vi "Write Display Settings 2 File.vi"(8 "error in":errorcluster, 11 "State":T6={"ImageSource"=enum."Camera", "IMAQdx Cam"=refnum, "WorkDir"=path "", "Image Name Prefix"="", "ROI"={"Global Rectangle"=[], "Contours"=[]}, "BG Image"=refnum, "Display Image"=refnum, "Display settings"={"Min. Thresh."=0.0, "X"=0.0, "Y"=0.0, "ShowLineout"=FALSE, "ScaleParts"=10, "ShowLegende"=FALSE, "Target Cross"=FALSE, "Centroid Cross"=FALSE, "Target color"=16777226, "Centroid color"=16711680, "calibr. mm/px"=0.0}, "Mask image"=refnum, "ConfigDir"=path "", "Display ref"=refnum, "Saved ROIs"=[], "Selected ROI"="", "Analyze Objects"=[], "Analysis Params"=variant, "Analysis Results"=variant, "Overlays?"=[], "Ref Palette type"=refnum, "Time in Filename?"=TRUE, "Save Report?"=TRUE, "Appl Params"=variant, "Show ZoomBtn?"=TRUE, "Image file"=path ""} {"ROI"."Contours"."Type" items=["No Selection", "Point", "Line", "Rectangle", "Oval", "Polygon", "Freehand Region", "Annulus", "Unused2", "Unused3", "Broken Line", "Freehand Line", "Rotated Rectangle"]}) -> (0 "error out":errorcluster, 3 "file path out":path)   [LabVIEW 2020, in "POLARIS IMAQ Display.xctl"]
doc: "Store some settings of POLARIS IMAQ Display to file. \n[in] State cluster of XControl\nVI maps paramters of interest to dummy controls like ROI, SavedROI, Display settings and calls \n\"save cotrol values.vi\". The dummy contorl must have the same names like dummy controls in Read Display Settings.vi\n\n\nauthor: Alexander Kessler, Helmholtz-Institut-Jena \nmaintainer: Alexander Kessler: alexander.kessler@uni-jena.de\n\n\n\nLicense Agreement for this software:\n\nCopyright (C)\nHelmholtz-Institut-Jena\nFröbelstieg 3\n07743 Jena\nGermany\n\nThis program is free software; you can redistribute it and/or modify it under the terms of the GNU General Public License as published by the Free Software Foundation; either version 2 of the license, or (at your option) any later version.\n\nThis program is distributed in the hope that it will be useful, but WITHOUT ANY WARRANTY; without even the implied warranty of MERCHANTABILITY or FITNESS FOR A PARTICULAR PURPOSE. See the GNU General License for more details (http://www.gnu.org)."
uses:
  POLARIS IMAQ Display.xctl
  State.ctl
  IMAQdx Cam/IMAQdx Cam.lvclass
  Properties/ImageSource.ctl
  <vilib>/vision/Image Controls.llb/IMAQ Image.ctl
  DisplaySettings.ctl
  Named ROI.ctl
  Analyze Classes/Analyze BaseClass/Analyze BaseClass.lvclass
  Palette.ctl
  Utility/POLARIS Vision utility.lvlib
panel:
  in  "Pallete":T1={"Teiler"=1, "Palette Type"=0} {"Teiler" min=1 max=5; "Palette Type" items=["Grayscale", "Binary", "Gradient", "Rainbow", "Temperature", "User Defined"]}
  in  "Zoom":cluster{"X":i32, "Y":i32}
  in  "Image Center":cluster{"X":u32, "Y":u32}
  out "Image":T2(plugin-control)
  in  "Display settings":T3={"Min. Thresh."=0.0, "X"=0.0, "Y"=0.0, "ShowLineout"=FALSE, "ScaleParts"=10, "ShowLegende"=FALSE, "Target Cross"=FALSE, "Centroid Cross"=FALSE, "Target color"=16777226, "Centroid color"=16711680, "calibr. mm/px"=0.0}
  in  "ROI":T4 {"Contours"."Type" items=["No Selection", "Point", "Line", "Rectangle", "Oval", "Polygon", "Freehand Region", "Annulus", "Unused2", "Unused3", "Broken Line", "Freehand Line", "Rotated Rectangle"]}
  in  "Saved ROIs":T5[](array[typedef])
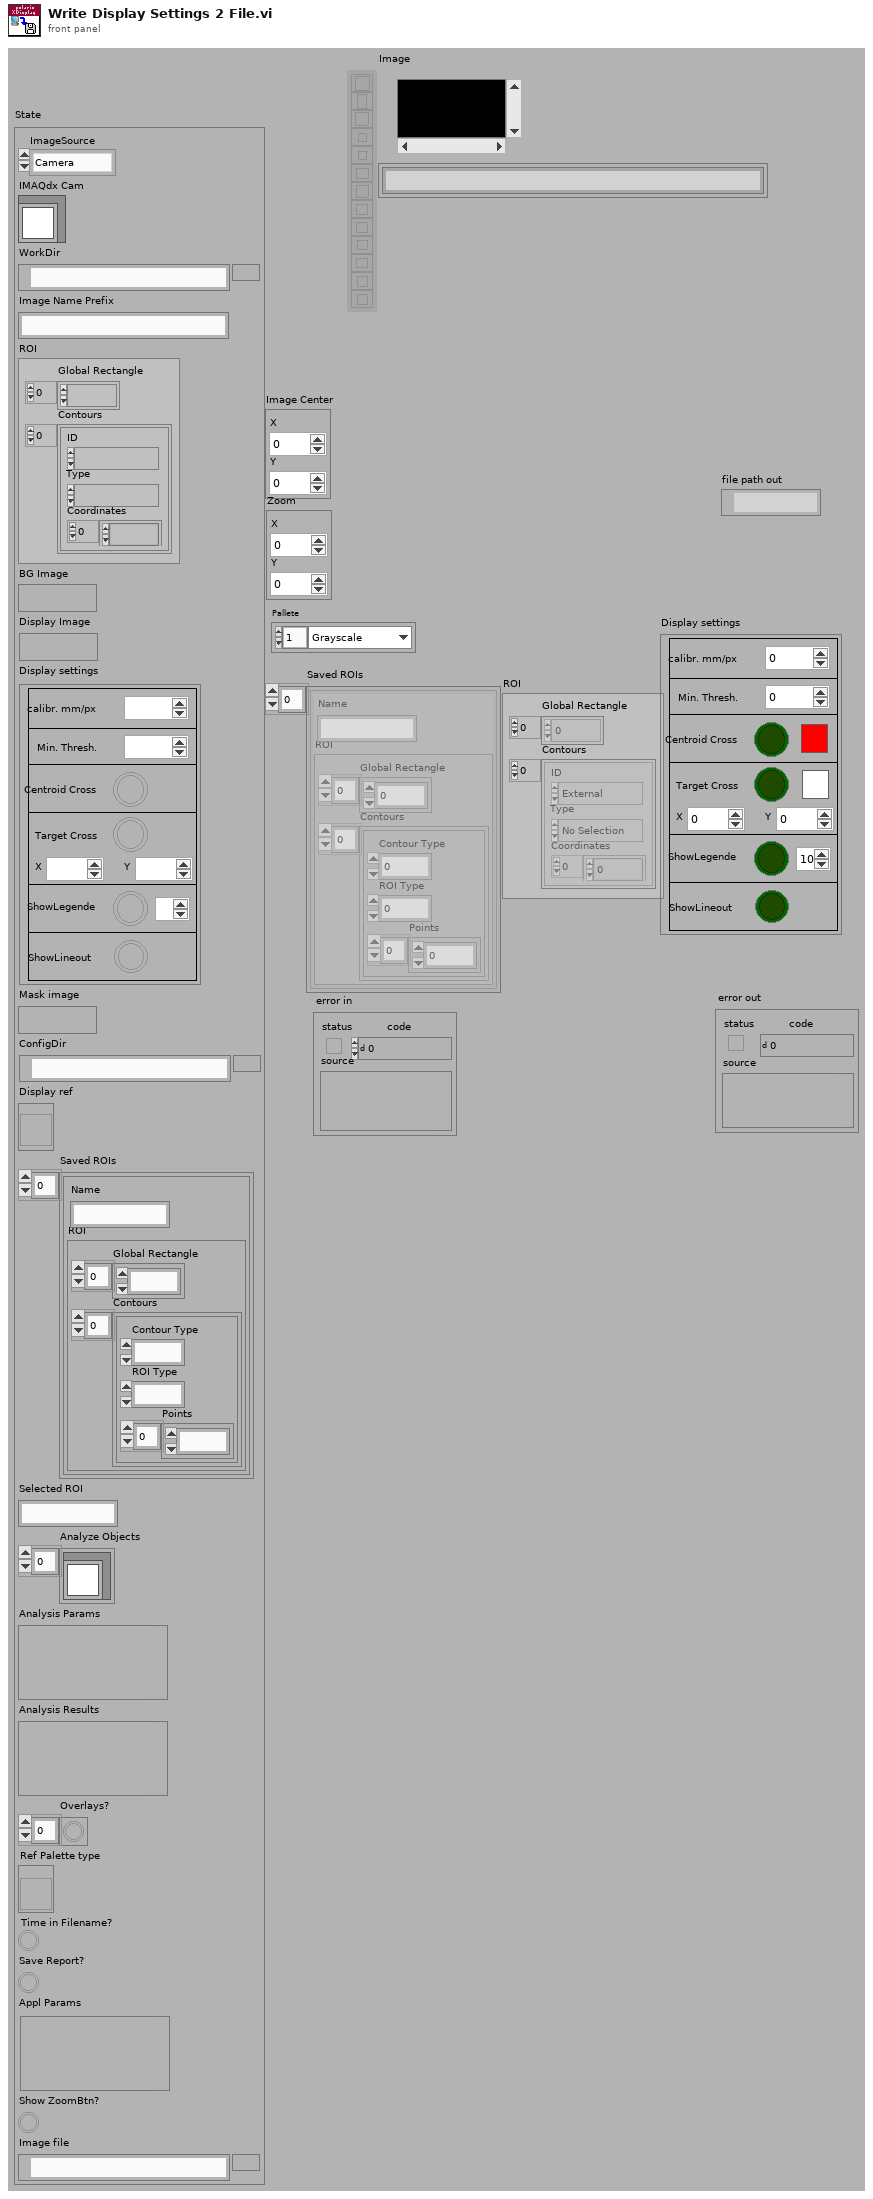
[diagram p1: front panel]
types:
  T1 = typedef "POLARIS IMAQ Display.xctl/Palette.ctl" = cluster{"Teiler":i32, "Palette Type":u32}
  T2 = typedef "IMAQ Image.ctl" = refnum<image>
  T3 = typedef "POLARIS IMAQ Display.xctl/DisplaySettings.ctl" = cluster{"Min. Thresh.":sgl, "X":dbl, "Y":dbl, "ShowLineout":bool, "ScaleParts":i32, "ShowLegende":bool, "Target Cross":bool, "Centroid Cross":bool, "Target color":u32, "Centroid color":u32, "calibr. mm/px":sgl}
  T4 = typedef "ROI Descriptor" = cluster{"Global Rectangle":i32[], "Contours":cluster{"ID":enum32{"External", "Internal"}, "Type":u32, "Coordinates":i32[]}[]}
  T5 = typedef "POLARIS IMAQ Display.xctl/Named ROI.ctl" = cluster{"ROI":cluster{"Global Rectangle":i32[], "Contours":cluster{"Contour Type":u32, "ROI Type":u32, "Points":i32[]}[]}, "Name":string}
  T6 = typedef "POLARIS IMAQ Display.xctl/State.ctl" = cluster{"ImageSource":T7, "IMAQdx Cam":refnum<class "IMAQdx Cam.lvclass">, "WorkDir":path, "Image Name Prefix":string, "ROI":T4, "BG Image":T2, "Display Image":T2, "Display settings":T3, "Mask image":T2, "ConfigDir":path, "Display ref":refnum<vi>, "Saved ROIs":T5[], "Selected ROI":string, "Analyze Objects":refnum<class "Analyze BaseClass.lvclass">[], "Analysis Params":variant, "Analysis Results":variant, "Overlays?":bool[], "Ref Palette type":refnum<vi>, "Time in Filename?":bool, "Save Report?":bool, "Appl Params":variant, "Show ZoomBtn?":bool, "Image file":path}
  T7 = typedef "POLARIS IMAQ Display.xctl/ImageSource.ctl" = enum16{"Camera", "File"}
  T8 = typedef "IMAQdx.ctl" = refnum<k21>
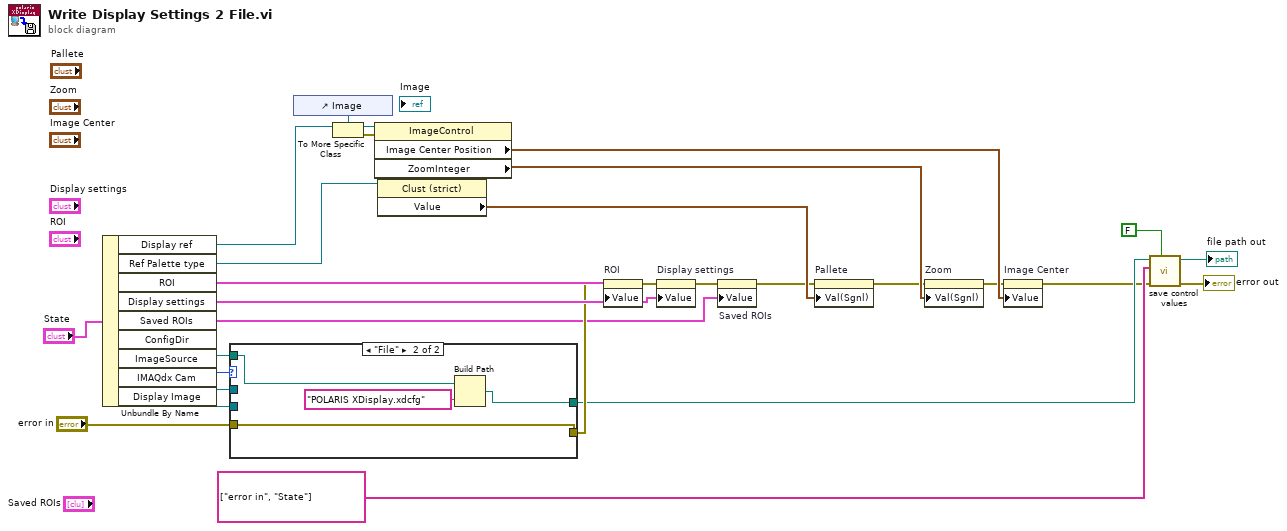
[diagram p0: block diagram]
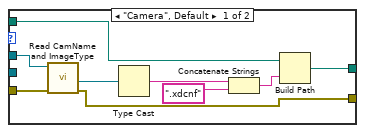
[diagram p2: hidden frame]
diagram:
  n1 = Unbundle By Name("State") -> ("Display ref"=w9:refnum<vi>, "Ref Palette type"=w4:refnum<vi>, "ROI"=w23:T4, "Display settings"=w22:T3, "Saved ROIs"=w13:T5[], "ConfigDir"=w17:path, "ImageSource"=w19:T7, "IMAQdx Cam"=w27:refnum<class "IMAQdx Cam.lvclass">, "Display Image"=w18:T2)
  n2 = case shown="\"File\"" w19 {
    tunnel: w27 -> [w38 _]
    tunnel: "error in" -> [w37 w42]
    tunnel: [w35 w42] -> w20
    tunnel: w18 -> [_ _]
    tunnel: w17 -> [w31 w41]
    tunnel: [w30 w39] -> w16
    frame "Camera", Default {
      n3 = call-dynamic "Read CamName and ImageType.vi"("error in (no error)"=w37, "IMAQdx Cam in"=w38) -> ("error out"=w35:errorcluster, "Camera"=w36:T8)  [unwired: 6 in, 2 out]
      n4 = Type Cast(x=w36) -> (*(type *) &x=w32:string)  [unwired: 1 in]
      n5 = Concatenate Strings(w32, ".xdcnf" ("string")) -> (w33:string)
      n6 = Build Path(base path=w31, name or relative path=w33) -> (appended path=w30:path)
    }
    frame "File" {
      n7 = Build Path(base path=w41, name or relative path="POLARIS XDisplay.xdcfg") -> (appended path=w39:path)
    }
  }
  n8 = control-ref of="Image"() -> (w10:refnum<vi>)
  n9 = To More Specific Class(target class=w10, reference=w9) -> (specific class reference=w11:refnum<vi>, error out=w12:errorcluster)  [unwired: 1 in]
  n10 = property class="ImageControl"(reference=w11, error in=w12) -> ("Image Center Position"=w7:cluster{"X":u32, "Y":u32}, "ZoomInteger"=w5:cluster{"X":i32, "Y":i32})  [unwired: 2 out]
  n11 = property class="Clust (strict)"(reference=w4) -> ("Value"=w3:T1)  [unwired: 1 in, 2 out]
  n12 = property on="ROI" class="Clust (strict)"(error in=w20, "Value"=w23) -> (error out=w21:errorcluster)  [unwired: 1 in, 1 out]
  n13 = property on="Display settings" class="Clust (strict)"(error in=w21, "Value"=w22) -> (error out=w14:errorcluster)  [unwired: 1 in, 1 out]
  n14 = property on="Saved ROIs" class="Arr (strict)"(error in=w14, "Value"=w13) -> (error out=w2:errorcluster)  [unwired: 1 in, 1 out]
  n15 = property on="Pallete" class="Clust (strict)"(error in=w2, "Val(Sgnl)"=w3) -> (error out=w1:errorcluster)  [unwired: 1 in, 1 out]
  n16 = property on="Zoom" class="Clust (strict)"(error in=w1, "Val(Sgnl)"=w5) -> (error out=w6:errorcluster)  [unwired: 1 in, 1 out]
  n17 = property on="Image Center" class="Clust (strict)"(error in=w6, "Value"=w7) -> (error out=w8:errorcluster)  [unwired: 1 in, 1 out]
  n18 = call "save control values.vi"("Append timestamp (true)"=FALSE, "error in"=w8, "Dont save"=string[] ["error in", "State"], "Path"=w16) -> ("error out"=→"error out":errorcluster, "file path out"=→"file path out":path)  [unwired: 4 in]
